vi "JoystickOpen.vi"(8 "error in (no error)":errorcluster, 11 "RobotConfigIn":T1={"Motors"={"RightDrivePrimary"={"CAN Address"=0, "Invert"=FALSE, "InvertSensor"=FALSE, "Unit Conversion Factor"=0.0, "Brake Mode"=enum."Override to Brake", "Reverse Limt Switch Mode"=enum."Disabled", "Forward Limt Swith Mode"=enum."Disabled", "PWM Channel"=enum."Invalid", "Motor Controller Type"=enum."Talon SRX", "Peak Current (A)"=0, "Continuous Current (A)"=0, "Peak Duration (ms)"=0, "Current Limit Enable"=FALSE}, "RightDriveSecondary"={"CAN Address"=0, "Invert"=FALSE, "InvertSensor"=FALSE, "Unit Conversion Factor"=0.0, "Brake Mode"=enum."Override to Brake", "Reverse Limt Switch Mode"=enum."Disabled", "Forward Limt Swith Mode"=enum."Disabled", "PWM Channel"=enum."Invalid", "Motor Controller Type"=enum."Talon SRX", "Peak Current (A)"=0, "Continuous Current (A)"=0, "Peak Duration (ms)"=0, "Current Limit Enable"=FALSE}, "LeftDrivePrimary"={"CAN Address"=0, "Invert"=FALSE, "InvertSensor"=FALSE, "Unit Conversion Factor"=0.0, "Brake Mode"=enum."Override to Brake", "Reverse Limt Switch Mode"=enum."Disabled", "Forward Limt Swith Mode"=enum."Disabled", "PWM Channel"=enum."Invalid", "Motor Controller Type"=enum."Talon SRX", "Peak Current (A)"=0, "Continuous Current (A)"=0, "Peak Duration (ms)"=0, "Current Limit Enable"=FALSE}, "LeftDriveSecondary"={"CAN Address"=0, "Invert"=FALSE, "InvertSensor"=FALSE, "Unit Conversion Factor"=0.0, "Brake Mode"=enum."Override to Brake", "Reverse Limt Switch Mode"=enum."Disabled", "Forward Limt Swith Mode"=enum."Disabled", "PWM Channel"=enum."Invalid", "Motor Controller Type"=enum."Talon SRX", "Peak Current (A)"=0, "Continuous Current (A)"=0, "Peak Duration (ms)"=0, "Current Limit Enable"=FALSE}, "RightShooter"={"CAN Address"=0, "Invert"=FALSE, "InvertSensor"=FALSE, "Unit Conversion Factor"=0.0, "Brake Mode"=enum."Override to Brake", "Reverse Limt Switch Mode"=enum."Disabled", "Forward Limt Swith Mode"=enum."Disabled", "PWM Channel"=enum."Invalid", "Motor Controller Type"=enum."Talon SRX", "Peak Current (A)"=0, "Continuous Current (A)"=0, "Peak Duration (ms)"=0, "Current Limit Enable"=FALSE}, "LeftShooter"={"CAN Address"=0, "Invert"=FALSE, "InvertSensor"=FALSE, "Unit Conversion Factor"=0.0, "Brake Mode"=enum."Override to Brake", "Reverse Limt Switch Mode"=enum."Disabled", "Forward Limt Swith Mode"=enum."Disabled", "PWM Channel"=enum."Invalid", "Motor Controller Type"=enum."Talon SRX", "Peak Current (A)"=0, "Continuous Current (A)"=0, "Peak Duration (ms)"=0, "Current Limit Enable"=FALSE}, "ShooterRotate"={"CAN Address"=0, "Invert"=FALSE, "InvertSensor"=FALSE, "Unit Conversion Factor"=0.0, "Brake Mode"=enum."Override to Brake", "Reverse Limt Switch Mode"=enum."Disabled", "Forward Limt Swith Mode"=enum."Disabled", "PWM Channel"=enum."Invalid", "Motor Controller Type"=enum."Talon SRX", "Peak Current (A)"=0, "Continuous Current (A)"=0, "Peak Duration (ms)"=0, "Current Limit Enable"=FALSE}, "ShooterHood"={"CAN Address"=0, "Invert"=FALSE, "InvertSensor"=FALSE, "Unit Conversion Factor"=0.0, "Brake Mode"=enum."Override to Brake", "Reverse Limt Switch Mode"=enum."Disabled", "Forward Limt Swith Mode"=enum."Disabled", "PWM Channel"=enum."Invalid", "Motor Controller Type"=enum."Talon SRX", "Peak Current (A)"=0, "Continuous Current (A)"=0, "Peak Duration (ms)"=0, "Current Limit Enable"=FALSE}, "HopperWheel"={"CAN Address"=0, "Invert"=FALSE, "InvertSensor"=FALSE, "Unit Conversion Factor"=0.0, "Brake Mode"=enum."Override to Brake", "Reverse Limt Switch Mode"=enum."Disabled", "Forward Limt Swith Mode"=enum."Disabled", "PWM Channel"=enum."Invalid", "Motor Controller Type"=enum."Talon SRX", "Peak Current (A)"=0, "Continuous Current (A)"=0, "Peak Duration (ms)"=0, "Current Limit Enable"=FALSE}, "Elevator"={"CAN Address"=0, "Invert"=FALSE, "InvertSensor"=FALSE, "Unit Conversion Factor"=0.0, "Brake Mode"=enum."Override to Brake", "Reverse Limt Switch Mode"=enum."Disabled", "Forward Limt Swith Mode"=enum."Disabled", "PWM Channel"=enum."Invalid", "Motor Controller Type"=enum."Talon SRX", "Peak Current (A)"=0, "Continuous Current (A)"=0, "Peak Duration (ms)"=0, "Current Limit Enable"=FALSE}, "ClimberRaise"={"CAN Address"=0, "Invert"=FALSE, "InvertSensor"=FALSE, "Unit Conversion Factor"=0.0, "Brake Mode"=enum."Override to Brake", "Reverse Limt Switch Mode"=enum."Disabled", "Forward Limt Swith Mode"=enum."Disabled", "PWM Channel"=enum."Invalid", "Motor Controller Type"=enum."Talon SRX", "Peak Current (A)"=0, "Continuous Current (A)"=0, "Peak Duration (ms)"=0, "Current Limit Enable"=FALSE}, "ClimberPullUp"={"CAN Address"=0, "Invert"=FALSE, "InvertSensor"=FALSE, "Unit Conversion Factor"=0.0, "Brake Mode"=enum."Override to Brake", "Reverse Limt Switch Mode"=enum."Disabled", "Forward Limt Swith Mode"=enum."Disabled", "PWM Channel"=enum."Invalid", "Motor Controller Type"=enum."Talon SRX", "Peak Current (A)"=0, "Continuous Current (A)"=0, "Peak Duration (ms)"=0, "Current Limit Enable"=FALSE}, "Intake"={"CAN Address"=0, "Invert"=FALSE, "InvertSensor"=FALSE, "Unit Conversion Factor"=0.0, "Brake Mode"=enum."Override to Brake", "Reverse Limt Switch Mode"=enum."Disabled", "Forward Limt Swith Mode"=enum."Disabled", "PWM Channel"=enum."Invalid", "Motor Controller Type"=enum."Talon SRX", "Peak Current (A)"=0, "Continuous Current (A)"=0, "Peak Duration (ms)"=0, "Current Limit Enable"=FALSE}, "ControlPanel"={"CAN Address"=0, "Invert"=FALSE, "InvertSensor"=FALSE, "Unit Conversion Factor"=0.0, "Brake Mode"=enum."Override to Brake", "Reverse Limt Switch Mode"=enum."Disabled", "Forward Limt Swith Mode"=enum."Disabled", "PWM Channel"=enum."Invalid", "Motor Controller Type"=enum."Talon SRX", "Peak Current (A)"=0, "Continuous Current (A)"=0, "Peak Duration (ms)"=0, "Current Limit Enable"=FALSE}}, "PID"={"Shooter"={"P"=0.0, "I"=0.0, "D"=0.0, "F"=0.0, "IZone"=0.0}, "Turret"={"P"=0.0, "I"=0.0, "D"=0.0, "F"=0.0, "IZone"=0.0}, "Elevator"={"P"=0.0, "I"=0.0, "D"=0.0, "F"=0.0, "IZone"=0.0}, "ControlPanel"={"P"=0.0, "I"=0.0, "D"=0.0, "F"=0.0, "IZone"=0.0}}, "MotionMagic"={"Turret"={"CruiseVelocity"=0, "Acceleration"=0}, "Elevator"={"CruiseVelocity"=0, "Acceleration"=0}, "ControlPanel"={"CruiseVelocity"=0, "Acceleration"=0}}, "Sensors"={"IMU"={"Yaw Axis"=enum."Z", "SPI Bus"=enum."SPI MXP", "AHRS Algorithm"=enum."Complementary", "Calibration Time (s)"=3.0, "Calibrate On Open"=TRUE}}, "Solenoids"={"Intake"={"SolenoidChannel"=enum."Solenoid 0", "Invert"=FALSE}}, "EnableCompressor"=FALSE, "RobotDimensions"={"Wheelbase(in)"=0.0, "Length(in)"=0.0}, "CameraMounting"={"LensHeight(in)"=0.0, "RotationRadius(in)"=0.0, "Pitch(deg)"=0.0}}) -> (0 "error out":errorcluster, 3 "RobotConfigOut":T1={"Motors"={"RightDrivePrimary"={"CAN Address"=0, "Invert"=FALSE, "InvertSensor"=FALSE, "Unit Conversion Factor"=0.0, "Brake Mode"=enum."Override to Brake", "Reverse Limt Switch Mode"=enum."Disabled", "Forward Limt Swith Mode"=enum."Disabled", "PWM Channel"=enum."Invalid", "Motor Controller Type"=enum."Talon SRX", "Peak Current (A)"=0, "Continuous Current (A)"=0, "Peak Duration (ms)"=0, "Current Limit Enable"=FALSE}, "RightDriveSecondary"={"CAN Address"=0, "Invert"=FALSE, "InvertSensor"=FALSE, "Unit Conversion Factor"=0.0, "Brake Mode"=enum."Override to Brake", "Reverse Limt Switch Mode"=enum."Disabled", "Forward Limt Swith Mode"=enum."Disabled", "PWM Channel"=enum."Invalid", "Motor Controller Type"=enum."Talon SRX", "Peak Current (A)"=0, "Continuous Current (A)"=0, "Peak Duration (ms)"=0, "Current Limit Enable"=FALSE}, "LeftDrivePrimary"={"CAN Address"=0, "Invert"=FALSE, "InvertSensor"=FALSE, "Unit Conversion Factor"=0.0, "Brake Mode"=enum."Override to Brake", "Reverse Limt Switch Mode"=enum."Disabled", "Forward Limt Swith Mode"=enum."Disabled", "PWM Channel"=enum."Invalid", "Motor Controller Type"=enum."Talon SRX", "Peak Current (A)"=0, "Continuous Current (A)"=0, "Peak Duration (ms)"=0, "Current Limit Enable"=FALSE}, "LeftDriveSecondary"={"CAN Address"=0, "Invert"=FALSE, "InvertSensor"=FALSE, "Unit Conversion Factor"=0.0, "Brake Mode"=enum."Override to Brake", "Reverse Limt Switch Mode"=enum."Disabled", "Forward Limt Swith Mode"=enum."Disabled", "PWM Channel"=enum."Invalid", "Motor Controller Type"=enum."Talon SRX", "Peak Current (A)"=0, "Continuous Current (A)"=0, "Peak Duration (ms)"=0, "Current Limit Enable"=FALSE}, "RightShooter"={"CAN Address"=0, "Invert"=FALSE, "InvertSensor"=FALSE, "Unit Conversion Factor"=0.0, "Brake Mode"=enum."Override to Brake", "Reverse Limt Switch Mode"=enum."Disabled", "Forward Limt Swith Mode"=enum."Disabled", "PWM Channel"=enum."Invalid", "Motor Controller Type"=enum."Talon SRX", "Peak Current (A)"=0, "Continuous Current (A)"=0, "Peak Duration (ms)"=0, "Current Limit Enable"=FALSE}, "LeftShooter"={"CAN Address"=0, "Invert"=FALSE, "InvertSensor"=FALSE, "Unit Conversion Factor"=0.0, "Brake Mode"=enum."Override to Brake", "Reverse Limt Switch Mode"=enum."Disabled", "Forward Limt Swith Mode"=enum."Disabled", "PWM Channel"=enum."Invalid", "Motor Controller Type"=enum."Talon SRX", "Peak Current (A)"=0, "Continuous Current (A)"=0, "Peak Duration (ms)"=0, "Current Limit Enable"=FALSE}, "ShooterRotate"={"CAN Address"=0, "Invert"=FALSE, "InvertSensor"=FALSE, "Unit Conversion Factor"=0.0, "Brake Mode"=enum."Override to Brake", "Reverse Limt Switch Mode"=enum."Disabled", "Forward Limt Swith Mode"=enum."Disabled", "PWM Channel"=enum."Invalid", "Motor Controller Type"=enum."Talon SRX", "Peak Current (A)"=0, "Continuous Current (A)"=0, "Peak Duration (ms)"=0, "Current Limit Enable"=FALSE}, "ShooterHood"={"CAN Address"=0, "Invert"=FALSE, "InvertSensor"=FALSE, "Unit Conversion Factor"=0.0, "Brake Mode"=enum."Override to Brake", "Reverse Limt Switch Mode"=enum."Disabled", "Forward Limt Swith Mode"=enum."Disabled", "PWM Channel"=enum."Invalid", "Motor Controller Type"=enum."Talon SRX", "Peak Current (A)"=0, "Continuous Current (A)"=0, "Peak Duration (ms)"=0, "Current Limit Enable"=FALSE}, "HopperWheel"={"CAN Address"=0, "Invert"=FALSE, "InvertSensor"=FALSE, "Unit Conversion Factor"=0.0, "Brake Mode"=enum."Override to Brake", "Reverse Limt Switch Mode"=enum."Disabled", "Forward Limt Swith Mode"=enum."Disabled", "PWM Channel"=enum."Invalid", "Motor Controller Type"=enum."Talon SRX", "Peak Current (A)"=0, "Continuous Current (A)"=0, "Peak Duration (ms)"=0, "Current Limit Enable"=FALSE}, "Elevator"={"CAN Address"=0, "Invert"=FALSE, "InvertSensor"=FALSE, "Unit Conversion Factor"=0.0, "Brake Mode"=enum."Override to Brake", "Reverse Limt Switch Mode"=enum."Disabled", "Forward Limt Swith Mode"=enum."Disabled", "PWM Channel"=enum."Invalid", "Motor Controller Type"=enum."Talon SRX", "Peak Current (A)"=0, "Continuous Current (A)"=0, "Peak Duration (ms)"=0, "Current Limit Enable"=FALSE}, "ClimberRaise"={"CAN Address"=0, "Invert"=FALSE, "InvertSensor"=FALSE, "Unit Conversion Factor"=0.0, "Brake Mode"=enum."Override to Brake", "Reverse Limt Switch Mode"=enum."Disabled", "Forward Limt Swith Mode"=enum."Disabled", "PWM Channel"=enum."Invalid", "Motor Controller Type"=enum."Talon SRX", "Peak Current (A)"=0, "Continuous Current (A)"=0, "Peak Duration (ms)"=0, "Current Limit Enable"=FALSE}, "ClimberPullUp"={"CAN Address"=0, "Invert"=FALSE, "InvertSensor"=FALSE, "Unit Conversion Factor"=0.0, "Brake Mode"=enum."Override to Brake", "Reverse Limt Switch Mode"=enum."Disabled", "Forward Limt Swith Mode"=enum."Disabled", "PWM Channel"=enum."Invalid", "Motor Controller Type"=enum."Talon SRX", "Peak Current (A)"=0, "Continuous Current (A)"=0, "Peak Duration (ms)"=0, "Current Limit Enable"=FALSE}, "Intake"={"CAN Address"=0, "Invert"=FALSE, "InvertSensor"=FALSE, "Unit Conversion Factor"=0.0, "Brake Mode"=enum."Override to Brake", "Reverse Limt Switch Mode"=enum."Disabled", "Forward Limt Swith Mode"=enum."Disabled", "PWM Channel"=enum."Invalid", "Motor Controller Type"=enum."Talon SRX", "Peak Current (A)"=0, "Continuous Current (A)"=0, "Peak Duration (ms)"=0, "Current Limit Enable"=FALSE}, "ControlPanel"={"CAN Address"=0, "Invert"=FALSE, "InvertSensor"=FALSE, "Unit Conversion Factor"=0.0, "Brake Mode"=enum."Override to Brake", "Reverse Limt Switch Mode"=enum."Disabled", "Forward Limt Swith Mode"=enum."Disabled", "PWM Channel"=enum."Invalid", "Motor Controller Type"=enum."Talon SRX", "Peak Current (A)"=0, "Continuous Current (A)"=0, "Peak Duration (ms)"=0, "Current Limit Enable"=FALSE}}, "PID"={"Shooter"={"P"=0.0, "I"=0.0, "D"=0.0, "F"=0.0, "IZone"=0.0}, "Turret"={"P"=0.0, "I"=0.0, "D"=0.0, "F"=0.0, "IZone"=0.0}, "Elevator"={"P"=0.0, "I"=0.0, "D"=0.0, "F"=0.0, "IZone"=0.0}, "ControlPanel"={"P"=0.0, "I"=0.0, "D"=0.0, "F"=0.0, "IZone"=0.0}}, "MotionMagic"={"Turret"={"CruiseVelocity"=0, "Acceleration"=0}, "Elevator"={"CruiseVelocity"=0, "Acceleration"=0}, "ControlPanel"={"CruiseVelocity"=0, "Acceleration"=0}}, "Sensors"={"IMU"={"Yaw Axis"=enum."Z", "SPI Bus"=enum."SPI MXP", "AHRS Algorithm"=enum."Complementary", "Calibration Time (s)"=3.0, "Calibrate On Open"=TRUE}}, "Solenoids"={"Intake"={"SolenoidChannel"=enum."Solenoid 0", "Invert"=FALSE}}, "EnableCompressor"=FALSE, "RobotDimensions"={"Wheelbase(in)"=0.0, "Length(in)"=0.0}, "CameraMounting"={"LensHeight(in)"=0.0, "RotationRadius(in)"=0.0, "Pitch(deg)"=0.0}})   [LabVIEW 2019]
uses:
  <vilib>/Rock Robotics/WPI/Joystick/WPI_JoystickDeviceEnum.ctl
  <vilib>/Rock Robotics/WPI/ThirdParty/Phoenix-LabVIEW/Motor Controller/Controls/CTRE_Phoenix_MotorControl_NeutralMode.ctl
  <vilib>/Rock Robotics/WPI/ThirdParty/Phoenix-LabVIEW/Motor Controller/Controls/CTRE_Phoenix_MotorControl_LimitSwitchNormal.ctl
  <vilib>/Rock Robotics/SystemInterfaces/DIO/FPGA_DIOPWMChannel.ctl
  ArgosLib/Config/ConfigComponents/TypeDefs/Config_MotorCtrlType.ctl
  ArgosLib/ArgosLib.lvlib
  ArgosLib/Config/ConfigComponents/TypeDefs/Config_Motor.ctl
  ArgosLib/Config/ConfigComponents/TypeDefs/Config_PIDParams.ctl
  ArgosLib/Config/ConfigComponents/TypeDefs/Config_MotionMagicParams.ctl
  <vilib>/Rock Robotics/SystemInterfaces/spilib/spi_bus.ctl
  ArgosLib/Config/ConfigComponents/TypeDefs/Config_IMU.ctl
  <vilib>/Rock Robotics/WPI/Solenoid/WPI_SolenoidChannel.ctl
  ArgosLib/Config/ConfigComponents/TypeDefs/Config_SingleSolenoid.ctl
  TypeDefs/ConfigComponents/Config_RobotDimensions.ctl
  TypeDefs/ConfigComponents/Config_CameraMounting.ctl
  TypeDefs/ConfigComponents/Config_Robot.ctl
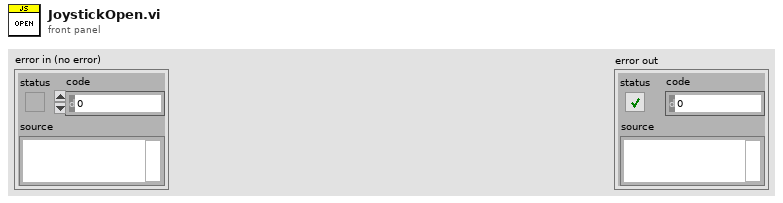
[diagram p1: front panel]
types:
  T1 = typedef "Config_Robot.ctl" = cluster{"Motors":cluster{"RightDrivePrimary":T2, "RightDriveSecondary":T2, "LeftDrivePrimary":T2, "LeftDriveSecondary":T2, "RightShooter":T2, "LeftShooter":T2, "ShooterRotate":T2, "ShooterHood":T2, "HopperWheel":T2, "Elevator":T2, "ClimberRaise":T2, "ClimberPullUp":T2, "Intake":T2, "ControlPanel":T2}, "PID":cluster{"Shooter":T7, "Turret":T7, "Elevator":T7, "ControlPanel":T7}, "MotionMagic":cluster{"Turret":T8, "Elevator":T8, "ControlPanel":T8}, "Sensors":cluster{"IMU":T9}, "Solenoids":cluster{"Intake":T11}, "EnableCompressor":bool, "RobotDimensions":T13, "CameraMounting":T14}
  T2 = typedef "ArgosLib.lvlib/Config_Motor.ctl" = cluster{"CAN Address":u8, "Invert":bool, "InvertSensor":bool, "Unit Conversion Factor":dbl, "Brake Mode":T3, "Reverse Limt Switch Mode":T4, "Forward Limt Swith Mode":T4, "PWM Channel":T5, "Motor Controller Type":T6, "Peak Current (A)":i32, "Continuous Current (A)":i32, "Peak Duration (ms)":i32, "Current Limit Enable":bool}
  T3 = typedef "CTRE_Phoenix_MotorControl_NeutralMode.ctl" = enum8{"EEPROMSetting", "Override to Coast", "Override to Brake"}
  T4 = typedef "CTRE_Phoenix_MotorControl_LimitSwitchNormal.ctl" = enum16{"Normally Open", "Normally Closed", "Disabled"}
  T5 = typedef "FPGA_DIOPWMChannel.ctl" = enum8{"PWM 0", "PWM 1", "PWM 2", "PWM 3", "PWM 4", "PWM 5", "PWM 6", "PWM 7", "PWM 8", "PWM 9", "PWM MXP 0", "PWM MXP 1", "PWM MXP 2", "PWM MXP 3", "PWM MXP 4", "PWM MXP 5", "PWM MXP 6", "PWM MXP 7", "PWM MXP 8", "PWM MXP 9", "Invalid"}
  T6 = typedef "ArgosLib.lvlib/Config_MotorCtrlType.ctl" = enum16{"Disabled", "Talon SRX", "Talon SR", "Venom", "Spark MAX"}
  T7 = typedef "ArgosLib.lvlib/Config_PIDParams.ctl" = cluster{"P":dbl, "I":dbl, "D":dbl, "F":dbl, "IZone":dbl}
  T8 = typedef "ArgosLib.lvlib/Config_MotionMagicParams.ctl" = cluster{"CruiseVelocity":i32, "Acceleration":i32}
  T9 = typedef "ArgosLib.lvlib/Config_IMU.ctl" = cluster{"Yaw Axis":enum16{"X", "Y", "Z"}, "SPI Bus":T10, "AHRS Algorithm":enum16{"Complementary", "Madgwick"}, "Calibration Time (s)":dbl, "Calibrate On Open":bool}
  T10 = typedef "spi_bus.ctl" = enum16{"SPI On-Board, CS0", "SPI On-Board, CS1", "SPI On-Board, CS2", "SPI On-Board, CS3", "SPI MXP", "Invalid"}
  T11 = typedef "ArgosLib.lvlib/Config_SingleSolenoid.ctl" = cluster{"SolenoidChannel":T12, "Invert":bool}
  T12 = typedef "WPI_SolenoidChannel.ctl" = enum8{"Solenoid 0", "Solenoid 1", "Solenoid 2", "Solenoid 3", "Solenoid 4", "Solenoid 5", "Solenoid 6", "Solenoid 7", "Invalid"}
  T13 = typedef "Config_RobotDimensions.ctl" = cluster{"Wheelbase(in)":dbl, "Length(in)":dbl}
  T14 = typedef "Config_CameraMounting.ctl" = cluster{"LensHeight(in)":dbl, "RotationRadius(in)":dbl, "Pitch(deg)":dbl}
  T15 = typedef "WPI_JoystickDeviceEnum.ctl" = enum16{"USB 0", "USB 1", "USB 2", "USB 3", "USB 4", "USB 5"}
  T16 = typedef "WPI_JoystickDevRef.ctl" = cluster{"Device":T15}
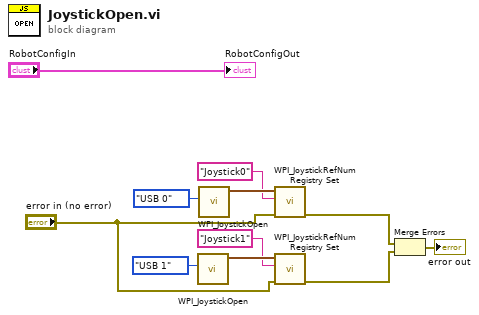
[diagram p0: block diagram]
diagram:
  n1 = call <vilib>:"WPI_JoystickOpen.vi"("JoystickDevice"=WPI_JoystickDeviceEnum."USB 1") -> ("JoystickDevRef"=w9:T16)  [unwired: 10 in]
  n2 = call <vilib>:"WPI_JoystickOpen.vi"("JoystickDevice"=WPI_JoystickDeviceEnum."USB 0") -> ("JoystickDevRef"=w10:T16)  [unwired: 10 in]
  n3 = call <vilib>:"WPI_JoystickRefNum Registry Set.vi"("error in (no error)"="error in (no error)", "refnum name"="Joystick0", "JoystickDevRef"=w10) -> ("error out"=w5:errorcluster)  [unwired: 7 in, 1 out]
  n4 = call <vilib>:"WPI_JoystickRefNum Registry Set.vi"("error in (no error)"="error in (no error)", "refnum name"="Joystick1", "JoystickDevRef"=w9) -> ("error out"=w4:errorcluster)  [unwired: 7 in, 1 out]
  n5 = Merge Errors(w5, w4) -> (→"error out":errorcluster)
  "RobotConfigOut" <- "RobotConfigIn"
